vi "Final Labview.vi"() -> ()   [LabVIEW 2021]
panel:
  out "Ball 5 Color":string
  out "ball 4 y":dbl
  out "Ball 4 Color":string
  out "ball 3 x":dbl
  out "ball 4 x":dbl
  out "ball 3 y":dbl
  out "Ball 3 Color":string
  out "ball 2 y":dbl
  out "ball 5 x":dbl
  out "Ball 2 Color":string
  out "ball 5 y":dbl
  out "ball 2 x":dbl
  out "Ball 1 Color":string
  out "ball 1 y":dbl
  out "ball 1 x":dbl
  in  "Display History":bool
  out "2D Picture":picture
  in  "Size of Rectangle":i16
  out "y2":dbl=769.0125 format="%#.9g"
  out "x2":dbl=769.0125 format="%#.9g"
  out "y1":dbl=769.0125 format="%#.9g"
  out "x1":dbl=769.0125 format="%#.9g"
  out "Color":dbl=769.0125 format="%#.9g"
  out "Case Number":dbl=769.0125 format="%#.9g"
  out "Y":dbl=769.0125 format="%#.9g"
  out "X":dbl=769.0125 format="%#.9g"
  in  "Input 8":dbl=769.0125 format="%#.9g"
  in  "Input 7":dbl=769.0125 format="%#.9g"
  in  "Input 6":dbl=769.0125 format="%#.9g"
  in  "Input 5":dbl=769.0125 format="%#.9g"
  in  "Input 4":dbl=769.0125 format="%#.9g"
  in  "Input 3":dbl=769.0125 format="%#.9g"
  in  "Input 2":dbl=769.0125 format="%#.9g"
  in  "Input":dbl=769.0125 format="%#.9g"
  in  "stop":bool
  in  "SEND Button":bool
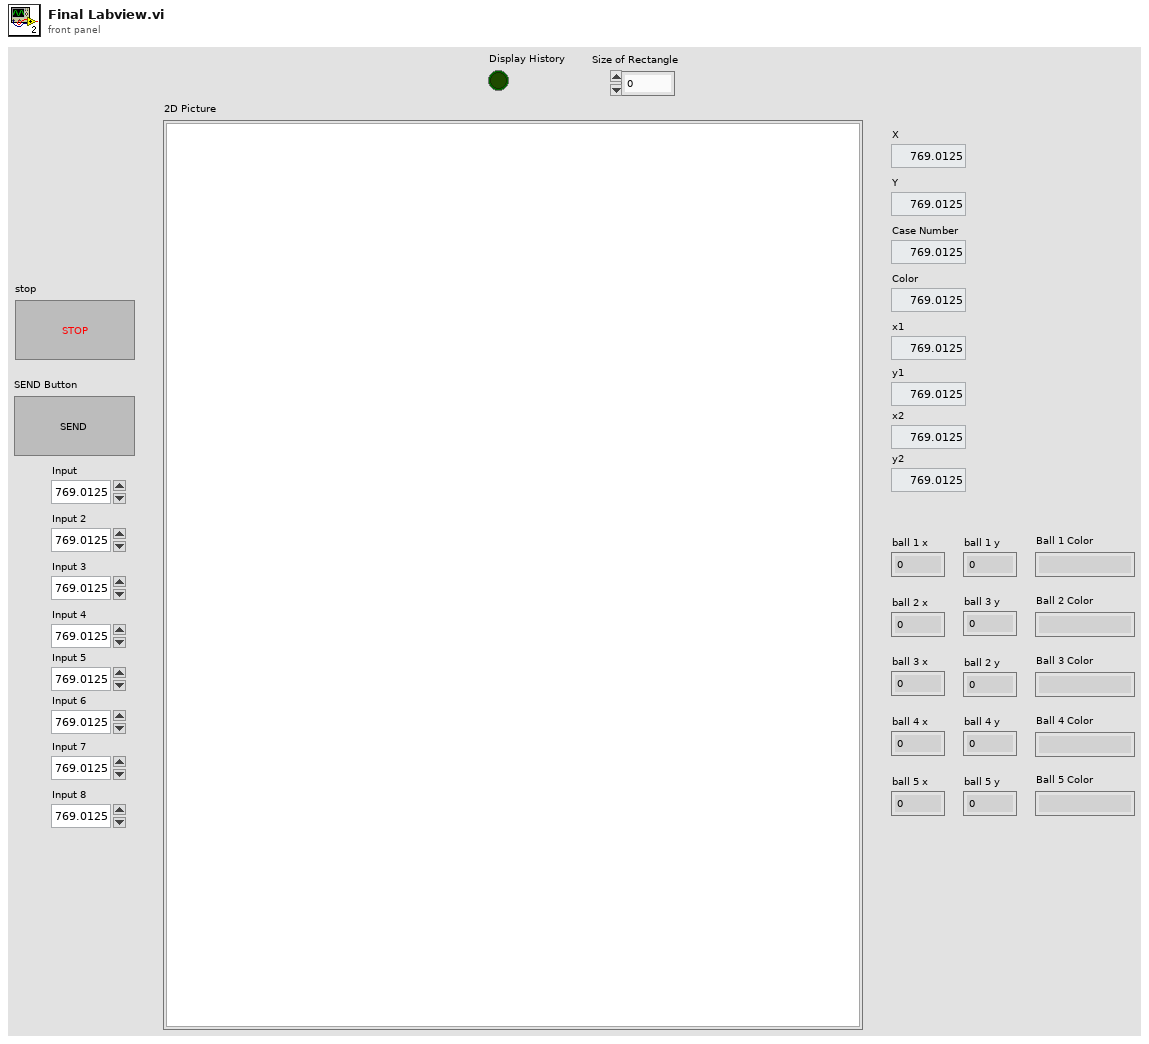
[diagram p1: front panel]
types:
  T1 = enum16{"Standard", "Buffered", "CRLF", "Immediate"}
  T2 = cluster{"Width":u16, "Style":enum32{"Solid", "Dash", "Dot", "DashDot", "DashDotDot"}}
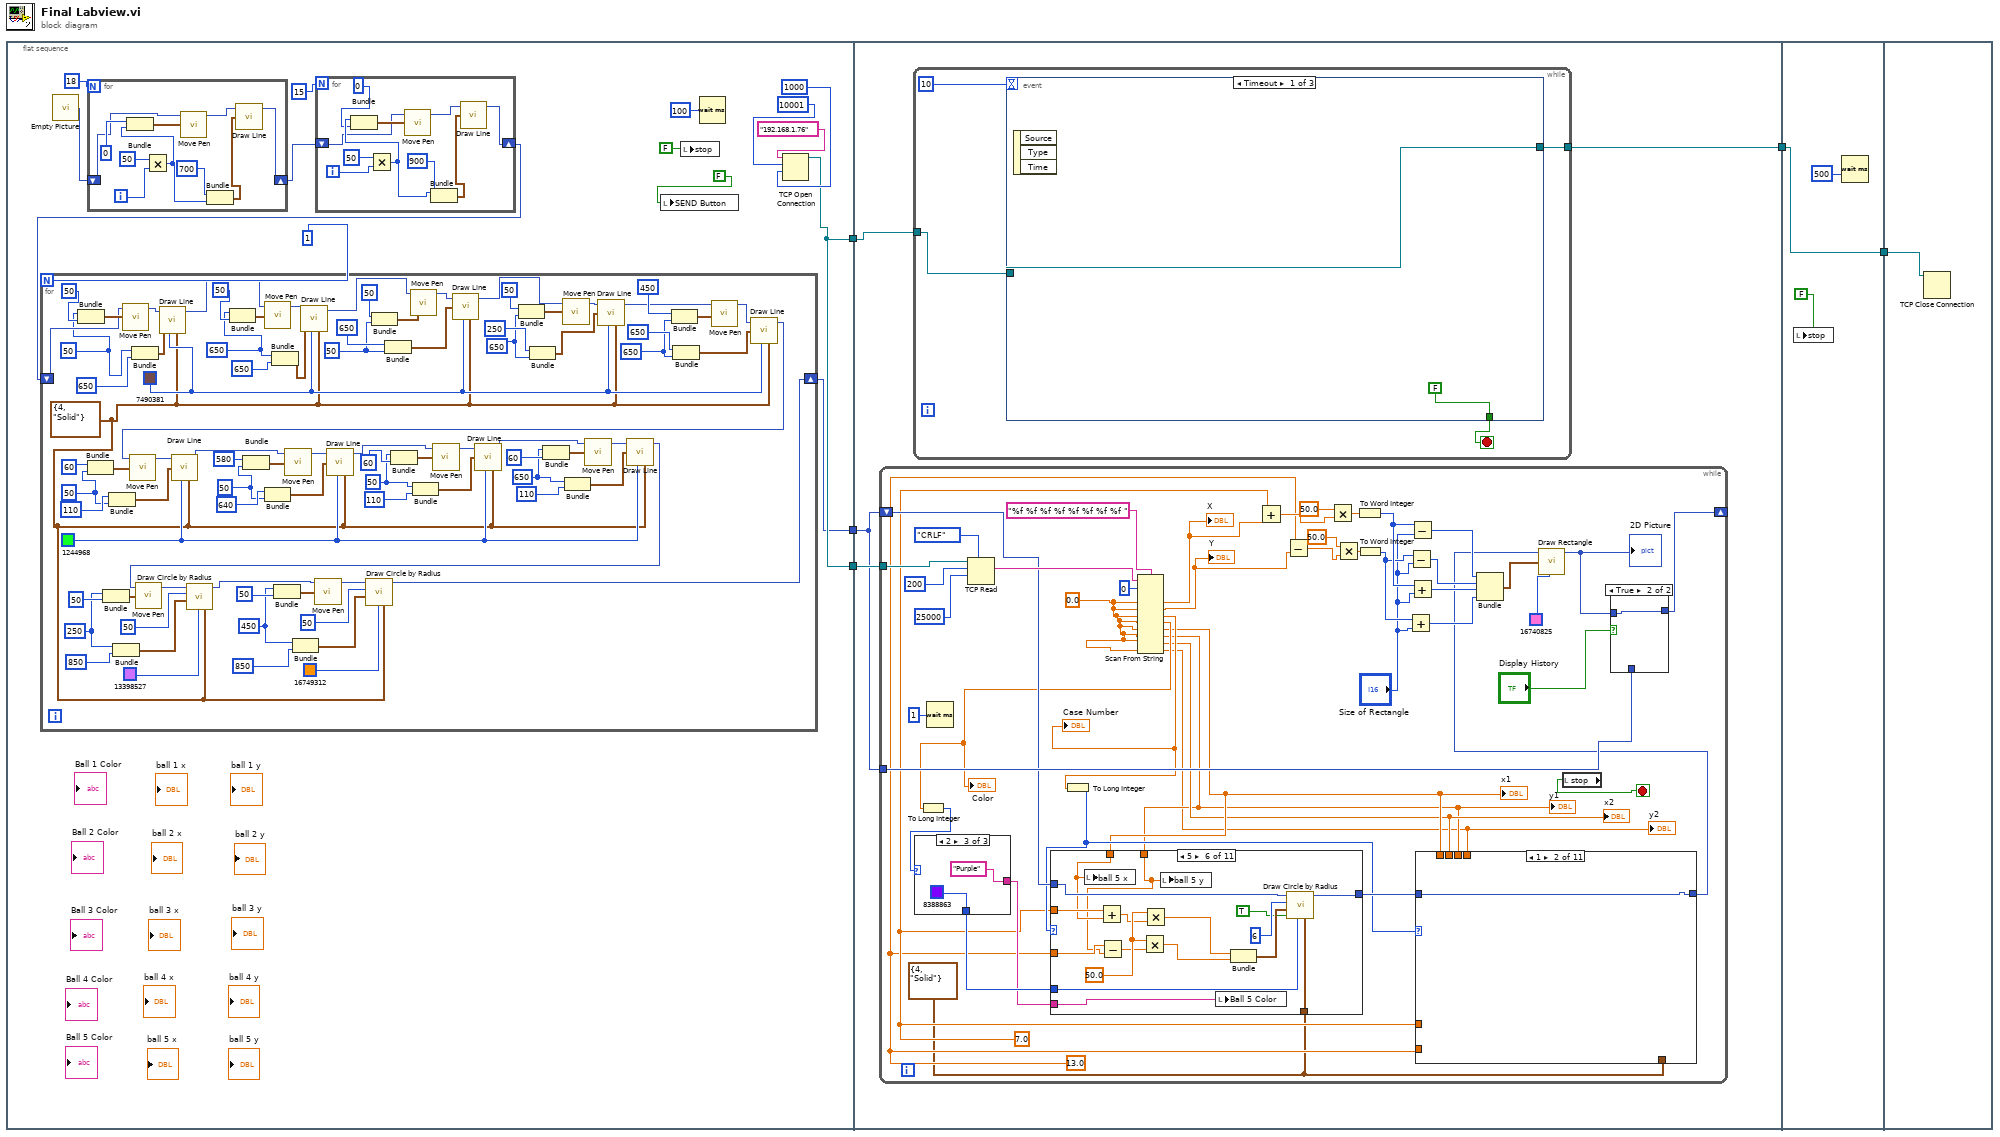
[diagram p0: block diagram]
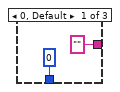
[diagram p2: hidden frame]
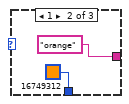
[diagram p3: hidden frame]
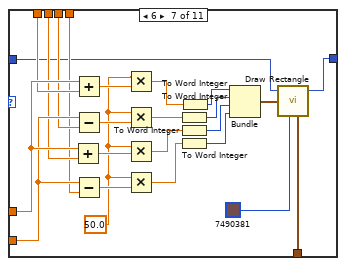
[diagram p9: hidden frame]
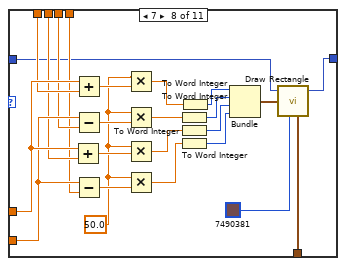
[diagram p10: hidden frame]
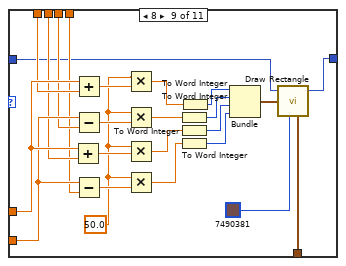
[diagram p11: hidden frame]
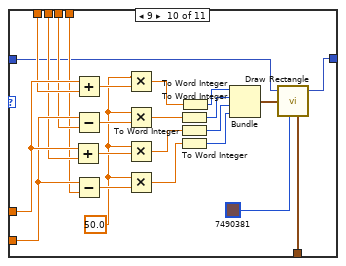
[diagram p12: hidden frame]
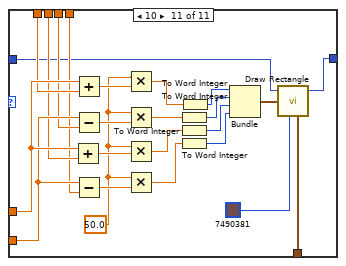
[diagram p13: hidden frame]
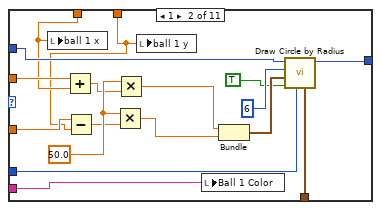
[diagram p15: hidden frame]
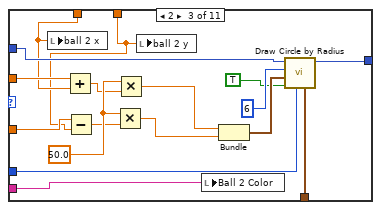
[diagram p16: hidden frame]
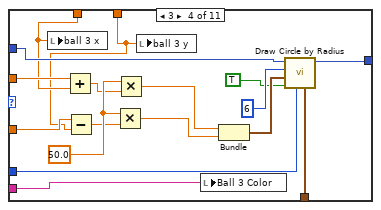
[diagram p17: hidden frame]
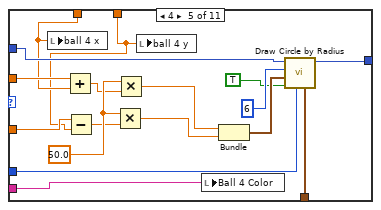
[diagram p18: hidden frame]
diagram:
  n1 = flat-sequence {
    tunnel: [w13] -> w5
    tunnel: [w13] -> w2
    tunnel: [w6] -> w1
    tunnel: w5 -> [w128]
    tunnel: [w127] -> w3
    tunnel: w2 -> [w126]
    tunnel: w1 -> [w125]
    tunnel: [w428] -> w4
    tunnel: w3 -> [w428]
    tunnel: w4 -> [w429]
    frame #0 {
      n2 = call "Empty Picture"() -> ("empty picture"=w9:picture)
      n3 = for {
        N: 18 -> [_]
        shift-right: [w115] -> w11
        shift-left: w9 -> [w116]
        i -> [w123]
        n4 = Multiply(x=50, y=w123) -> (x*y=w119:i32)
        n5 = Bundle(0, w119) -> (w120:cluster{i32, i32})  [unwired: 1 in]
        n6 = call <vilib>:"Move Pen.vi"("new position"=w120, "picture"=w116) -> ("new picture"=w124:picture)  [unwired: 3 in]
        n7 = Bundle(700, w119) -> (w117:cluster{i32, i32})  [unwired: 1 in]
        n8 = call <vilib>:"Draw Line.vi"("picture"=w124, "end point"=w117) -> ("new picture"=w115:picture)  [unwired: 7 in]
      }
      n9 = for {
        N: 15 -> [_]
        shift-right: [w105] -> w7
        shift-left: w11 -> [w106]
        i -> [w113]
        n10 = Multiply(x=50, y=w113) -> (x*y=w108:i32)
        n11 = Bundle(w108, 0) -> (w111:cluster{i32, i32})  [unwired: 1 in]
        n12 = call <vilib>:"Move Pen.vi"("new position"=w111, "picture"=w106) -> ("new picture"=w114:picture)  [unwired: 3 in]
        n13 = Bundle(w108, 900) -> (w110:cluster{i32, i32})  [unwired: 1 in]
        n14 = call <vilib>:"Draw Line.vi"("picture"=w114, "end point"=w110) -> ("new picture"=w105:picture)  [unwired: 7 in]
      }
      n15 = for {
        N: 1 -> [_]
        shift-right: [w21] -> w6
        shift-left: w7 -> [w99]
        w24 = 450 ("x")
        w32 = 250 ("x")
        w40 = 650 ("x")
        w42 = 50 ("x")
        w57 = 50 ("x")
        w46 = u32 1244968 ("Hilite")
        w63 = 50 ("x")
        w69 = 650 ("x")
        w20 = T2 {"Width"=4, "Style"=enum."Solid"} ("pen")
        w70 = 650 ("x")
        w71 = 50 ("x")
        w72 = 650 ("x")
        w74 = u32 7490381 ("Hilite")
        w73 = 50 ("x")
        n16 = Bundle("x"=w73, 50) -> (w103:cluster{"x":i32, i32})  [unwired: 1 in]
        n17 = Bundle(60, "x"=w63) -> (w66:cluster{i32, "x":i32})  [unwired: 1 in]
        n18 = Bundle("x"=w32, 50) -> (w39:cluster{"x":i32, i32})  [unwired: 1 in]
        n19 = Bundle(110, "x"=w63) -> (w64:cluster{i32, "x":i32})  [unwired: 1 in]
        n20 = Bundle("x"=w32, 850) -> (w33:cluster{"x":i32, i32})  [unwired: 1 in]
        n21 = call <vilib>:"Move Pen.vi"("new position"=w103, "picture"=w99) -> ("new picture"=w104:picture)  [unwired: 3 in]
        n22 = Bundle("x"=w73, 650) -> (w102:cluster{"x":i32, i32})  [unwired: 1 in]
        n23 = call <vilib>:"Draw Line.vi"("picture"=w104, "end point"=w102, "color(black)"=w74, "pen"=w20) -> ("new picture"=w93:picture)  [unwired: 5 in]
        n24 = Bundle("x"=w72, 50) -> (w97:cluster{"x":i32, i32})  [unwired: 1 in]
        n25 = Bundle(580, "x"=w57) -> (w60:cluster{i32, "x":i32})  [unwired: 1 in]
        n26 = call <vilib>:"Move Pen.vi"("new position"=w97, "picture"=w93) -> ("new picture"=w98:picture)  [unwired: 3 in]
        n27 = Bundle(640, "x"=w57) -> (w58:cluster{i32, "x":i32})  [unwired: 1 in]
        n28 = Bundle("x"=w72, 650) -> (w96:cluster{"x":i32, i32})  [unwired: 1 in]
        n29 = Bundle("x"=w24, 50) -> (w31:cluster{"x":i32, i32})  [unwired: 1 in]
        n30 = Bundle("x"=w24, 850) -> (w25:cluster{"x":i32, i32})  [unwired: 1 in]
        n31 = call <vilib>:"Draw Line.vi"("picture"=w98, "end point"=w96, "color(black)"=w74, "pen"=w20) -> ("new picture"=w89:picture)  [unwired: 5 in]
        n32 = Bundle(50, "x"=w71) -> (w91:cluster{i32, "x":i32})  [unwired: 1 in]
        n33 = Bundle(650, "x"=w71) -> (w90:cluster{i32, "x":i32})  [unwired: 1 in]
        n34 = Bundle("x"=w42, 60) -> (w55:cluster{"x":i32, i32})  [unwired: 1 in]
        n35 = call <vilib>:"Move Pen.vi"("new position"=w91, "picture"=w89) -> ("new picture"=w92:picture)  [unwired: 3 in]
        n36 = Bundle("x"=w42, 110) -> (w54:cluster{"x":i32, i32})  [unwired: 1 in]
        n37 = call <vilib>:"Draw Line.vi"("picture"=w92, "end point"=w90, "color(black)"=w74, "pen"=w20) -> ("new picture"=w84:picture)  [unwired: 5 in]
        n38 = Bundle(50, "x"=w70) -> (w86:cluster{i32, "x":i32})  [unwired: 1 in]
        n39 = Bundle(250, "x"=w70) -> (w85:cluster{i32, "x":i32})  [unwired: 1 in]
        n40 = Bundle("x"=w40, 60) -> (w52:cluster{"x":i32, i32})  [unwired: 1 in]
        n41 = call <vilib>:"Move Pen.vi"("new position"=w86, "picture"=w84) -> ("new picture"=w87:picture)  [unwired: 3 in]
        n42 = Bundle("x"=w40, 110) -> (w51:cluster{"x":i32, i32})  [unwired: 1 in]
        n43 = call <vilib>:"Draw Line.vi"("picture"=w87, "end point"=w85, "color(black)"=w74, "pen"=w20) -> ("new picture"=w75:picture)  [unwired: 5 in]
        n44 = Bundle(450, "x"=w69) -> (w79:cluster{i32, "x":i32})  [unwired: 1 in]
        n45 = Bundle(650, "x"=w69) -> (w78:cluster{i32, "x":i32})  [unwired: 1 in]
        n46 = call <vilib>:"Move Pen.vi"("new position"=w79, "picture"=w75) -> ("new picture"=w80:picture)  [unwired: 3 in]
        n47 = call <vilib>:"Draw Line.vi"("picture"=w80, "end point"=w78, "color(black)"=w74, "pen"=w20) -> ("new picture"=w50:picture)  [unwired: 5 in]
        n48 = call <vilib>:"Move Pen.vi"("new position"=w66, "picture"=w50) -> ("new picture"=w68:picture)  [unwired: 3 in]
        n49 = call <vilib>:"Draw Line.vi"("picture"=w68, "end point"=w64, "color(black)"=w46, "pen"=w20) -> ("new picture"=w49:picture)  [unwired: 5 in]
        n50 = call <vilib>:"Move Pen.vi"("new position"=w60, "picture"=w49) -> ("new picture"=w62:picture)  [unwired: 3 in]
        n51 = call <vilib>:"Draw Line.vi"("picture"=w62, "end point"=w58, "color(black)"=w46, "pen"=w20) -> ("new picture"=w48:picture)  [unwired: 5 in]
        n52 = call <vilib>:"Move Pen.vi"("new position"=w55, "picture"=w48) -> ("new picture"=w56:picture)  [unwired: 3 in]
        n53 = call <vilib>:"Draw Line.vi"("picture"=w56, "end point"=w54, "color(black)"=w46, "pen"=w20) -> ("new picture"=w47:picture)  [unwired: 5 in]
        n54 = call <vilib>:"Move Pen.vi"("new position"=w52, "picture"=w47) -> ("new picture"=w53:picture)  [unwired: 3 in]
        n55 = call <vilib>:"Draw Line.vi"("picture"=w53, "end point"=w51, "color(black)"=w46, "pen"=w20) -> ("new picture"=w23:picture)  [unwired: 5 in]
        n56 = call <vilib>:"Move Pen.vi"("new position"=w39, "picture"=w23) -> ("new picture"=w36:picture)  [unwired: 3 in]
        n57 = call <vilib>:"Draw Circle by Radius.vi"("pen"=w20, "color(black)"=u32 13398527 ("Hilite"), "pixel center"=w33, "radius"=i16 50, "picture"=w36) -> ("new picture"=w22:picture)  [unwired: 6 in]
        n58 = call <vilib>:"Move Pen.vi"("new position"=w31, "picture"=w22) -> ("new picture"=w28:picture)  [unwired: 3 in]
        n59 = call <vilib>:"Draw Circle by Radius.vi"("pen"=w20, "color(black)"=u32 16749312 ("Hilite"), "pixel center"=w25, "radius"=i16 50, "picture"=w28) -> ("new picture"=w21:picture)  [unwired: 6 in]
      }
      n60 = local write "SEND Button"(FALSE ("SEND Button")) -> ()
      n61 = local write "stop"(FALSE ("stop")) -> ()
      n62 = Wait (ms)(milliseconds to wait=u32 100) -> ()  [unwired: 1 out]
      n63 = TCP Open Connection(address="192.168.1.76", remote port or service name=u16 10001, timeout ms (60000)=1000) -> (connection ID=w13:refnum<k5>)  [unwired: 2 in, 1 out]
    }
    frame #1 {
      n64 = while {
        tunnel: w126 -> [w158]
        tunnel: w125 -> [w146]
        shift-right: [w155] -> _
        shift-left: w125 -> [w141]
        stop <- w147 stop-if-true
        w129 = T2 {"Width"=4, "Style"=enum."Solid"} ("pen")
        w134 = 13.0 ("x")
        w135 = 7.0 ("x")
        w145 = 0.0 ("default value 1")
        n65 = Wait (ms)(milliseconds to wait=u32 1) -> ()  [unwired: 1 out]
        n66 = TCP Read(connection ID=w158, bytes to read=200, 7:T1."CRLF" ("mode (standard)"), 9:25000 ("timeout ms (25000)")) -> (data out=w170:string)  [unwired: 1 in, 2 out]
        n67 = Scan From String(format string="%f %f %f %f %f %f %f %f ", input string=w170, initial scan location=u32 0, default 1=w145, default 2=w145, default 3=w145, default 4=w145, default 5=w145, default 6=w145, default 7=w145, default 8=w145) -> (output 1=w169:dbl, output 2=w168:dbl, output 3=w144:dbl, output 4=w138:dbl, output 5=w133:dbl, output 6=w131:dbl, output 7=w132:dbl, output 8=w130:dbl)  [unwired: 1 in, 3 out]
        "X" <- w169
        "Y" <- w168
        "Case Number" <- w144
        "Color" <- w138
        "x1" <- w133
        "y1" <- w131
        "x2" <- w132
        "y2" <- w130
        n68 = To Long Integer(number=w138) -> (32bit integer=w137:i32)
        n69 = case shown="2" w137 {
          tunnel: [u32 0 ("Hilite") u32 16749312 ("Hilite") u32 8388863 ("Hilite")] -> w143
          tunnel: ["" ("color 1") "orange" ("color 1") "Purple" ("color 1")] -> w142
          frame 0, Default {
          }
          frame 1 {
          }
          frame 2 {
          }
        }
        n70 = To Long Integer(number=w144) -> (32bit integer=w136:i32)
        n71 = case shown="5" w136 {
          tunnel: w141 -> [w308 w319 w336 w353 w370 w387 w394 w395 w396 w397 w398]
          tunnel: w131 -> [_ w313 w330 w347 w364 w381 _ _ _ _ _]
          tunnel: w133 -> [_ w314 w331 w348 w365 w382 _ _ _ _ _]
          tunnel: w129 -> [_ w322 w339 w356 w373 w390 _ _ _ _ _]
          tunnel: w143 -> [_ w321 w338 w355 w372 w389 _ _ _ _ _]
          tunnel: w142 -> [_ w320 w337 w354 w371 w388 _ _ _ _ _]
          tunnel: [w308 w318 w335 w352 w369 w386 w394 w395 w396 w397 w398] -> w140
          tunnel: w135 -> [_ w316 w333 w350 w367 w384 _ _ _ _ _]
          tunnel: w134 -> [_ w315 w332 w349 w366 w383 _ _ _ _ _]
          frame 0, Default {
          }
          frame 1 {
            w317 = 50.0 ("x")
            n72 = local write "ball 1 x"(w314) -> ()
            n73 = Add(x=w316, y=w314) -> (x+y=w312:dbl)
            n74 = Subtract(x=w315, y=w313) -> (x-y=w311:dbl)
            n75 = Multiply(x=w317, y=w311) -> (x*y=w309:dbl)
            n76 = Multiply(x=w317, y=w312) -> (x*y=w310:dbl)
            n77 = local write "ball 1 y"(w313) -> ()
            n78 = local write "Ball 1 Color"(w320) -> ()
            n79 = Bundle(w310, w309) -> (w324:cluster{dbl, dbl})  [unwired: 1 in]
            n80 = call <vilib>:"Draw Circle by Radius.vi"("pen"=w322, "color(black)"=w321, "fill?(F)"=TRUE, "pixel center"=w324, "radius"=i16 6, "picture"=w319) -> ("new picture"=w318:picture)  [unwired: 5 in]
          }
          frame 2 {
            w334 = 50.0 ("x")
            n81 = local write "ball 2 x"(w331) -> ()
            n82 = Add(x=w333, y=w331) -> (x+y=w329:dbl)
            n83 = Subtract(x=w332, y=w330) -> (x-y=w328:dbl)
            n84 = Multiply(x=w334, y=w328) -> (x*y=w326:dbl)
            n85 = Multiply(x=w334, y=w329) -> (x*y=w327:dbl)
            n86 = local write "ball 2 y"(w330) -> ()
            n87 = local write "Ball 2 Color"(w337) -> ()
            n88 = Bundle(w327, w326) -> (w341:cluster{dbl, dbl})  [unwired: 1 in]
            n89 = call <vilib>:"Draw Circle by Radius.vi"("pen"=w339, "color(black)"=w338, "fill?(F)"=TRUE, "pixel center"=w341, "radius"=i16 6, "picture"=w336) -> ("new picture"=w335:picture)  [unwired: 5 in]
          }
          frame 3 {
            w351 = 50.0 ("x")
            n90 = local write "ball 3 x"(w348) -> ()
            n91 = Add(x=w350, y=w348) -> (x+y=w346:dbl)
            n92 = Subtract(x=w349, y=w347) -> (x-y=w345:dbl)
            n93 = Multiply(x=w351, y=w345) -> (x*y=w343:dbl)
            n94 = Multiply(x=w351, y=w346) -> (x*y=w344:dbl)
            n95 = local write "ball 3 y"(w347) -> ()
            n96 = local write "Ball 3 Color"(w354) -> ()
            n97 = Bundle(w344, w343) -> (w358:cluster{dbl, dbl})  [unwired: 1 in]
            n98 = call <vilib>:"Draw Circle by Radius.vi"("pen"=w356, "color(black)"=w355, "fill?(F)"=TRUE, "pixel center"=w358, "radius"=i16 6, "picture"=w353) -> ("new picture"=w352:picture)  [unwired: 5 in]
          }
          frame 4 {
            w368 = 50.0 ("x")
            n99 = local write "ball 4 x"(w365) -> ()
            n100 = Add(x=w367, y=w365) -> (x+y=w363:dbl)
            n101 = Subtract(x=w366, y=w364) -> (x-y=w362:dbl)
            n102 = Multiply(x=w368, y=w362) -> (x*y=w360:dbl)
            n103 = Multiply(x=w368, y=w363) -> (x*y=w361:dbl)
            n104 = local write "ball 4 y"(w364) -> ()
            n105 = local write "Ball 4 Color"(w371) -> ()
            n106 = Bundle(w361, w360) -> (w375:cluster{dbl, dbl})  [unwired: 1 in]
            n107 = call <vilib>:"Draw Circle by Radius.vi"("pen"=w373, "color(black)"=w372, "fill?(F)"=TRUE, "pixel center"=w375, "radius"=i16 6, "picture"=w370) -> ("new picture"=w369:picture)  [unwired: 5 in]
          }
          frame 5 {
            w385 = 50.0 ("x")
            n108 = local write "ball 5 x"(w382) -> ()
            n109 = Add(x=w384, y=w382) -> (x+y=w380:dbl)
            n110 = Subtract(x=w383, y=w381) -> (x-y=w379:dbl)
            n111 = Multiply(x=w385, y=w379) -> (x*y=w377:dbl)
            n112 = Multiply(x=w385, y=w380) -> (x*y=w378:dbl)
            n113 = local write "ball 5 y"(w381) -> ()
            n114 = local write "Ball 5 Color"(w388) -> ()
            n115 = Bundle(w378, w377) -> (w392:cluster{dbl, dbl})  [unwired: 1 in]
            n116 = call <vilib>:"Draw Circle by Radius.vi"("pen"=w390, "color(black)"=w389, "fill?(F)"=TRUE, "pixel center"=w392, "radius"=i16 6, "picture"=w387) -> ("new picture"=w386:picture)  [unwired: 5 in]
          }
          frame 6 {
          }
          frame 7 {
          }
          frame 8 {
          }
          frame 9 {
          }
          frame 10 {
          }
        }
        n117 = Add(x=w135, y=w169) -> (x+y=w165:dbl)
        n118 = Subtract(x=w134, y=w168) -> (x-y=w164:dbl)
        n119 = Multiply(x=50.0, y=w165) -> (x*y=w162:dbl)
        n120 = Multiply(x=50.0, y=w164) -> (x*y=w163:dbl)
        n121 = To Word Integer(number=w162) -> (16bit integer=w161:i16)
        n122 = To Word Integer(number=w163) -> (16bit integer=w160:i16)
        n123 = Add(x=w160, y="Size of Rectangle") -> (x+y=w151:i16)
        n124 = Subtract(x=w160, y="Size of Rectangle") -> (x-y=w153:i16)
        n125 = Subtract(x=w161, y="Size of Rectangle") -> (x-y=w154:i16)
        n126 = Add(x=w161, y="Size of Rectangle") -> (x+y=w152:i16)
        n127 = case shown="1" w136 {
          tunnel: w140 -> [w182 w183 w184 w185 w186 w187 w196 w220 w244 w268 w292]
          tunnel: [w182 w183 w184 w185 w186 w187 w190 w214 w238 w262 w286] -> w139
          tunnel: w135 -> [_ _ _ _ _ _ w211 w235 w259 w283 w307]
          tunnel: w134 -> [_ _ _ _ _ _ w210 w234 w258 w282 w306]
          tunnel: w133 -> [_ _ _ _ _ _ w209 w233 w257 w281 w305]
          tunnel: w132 -> [_ _ _ _ _ _ w208 w232 w256 w280 w304]
          tunnel: w131 -> [_ _ _ _ _ _ w207 w231 w255 w279 w303]
          tunnel: w130 -> [_ _ _ _ _ _ w206 w230 w254 w278 w302]
          tunnel: w129 -> [_ _ _ _ _ _ w188 w212 w236 w260 w284]
          frame 0, Default {
          }
          frame 1 {
          }
          frame 2 {
          }
          frame 3 {
          }
          frame 4 {
          }
          frame 5 {
          }
          frame 6 {
            w201 = 50.0 ("x")
            n128 = Add(x=w211, y=w208) -> (x+y=w203:dbl)
            n129 = Add(x=w211, y=w209) -> (x+y=w205:dbl)
            n130 = Subtract(x=w210, y=w207) -> (x-y=w204:dbl)
            n131 = Subtract(x=w210, y=w206) -> (x-y=w202:dbl)
            n132 = Multiply(x=w201, y=w205) -> (x*y=w200:dbl)
            n133 = Multiply(x=w201, y=w204) -> (x*y=w199:dbl)
            n134 = Multiply(x=w201, y=w203) -> (x*y=w198:dbl)
            n135 = Multiply(x=w201, y=w202) -> (x*y=w197:dbl)
            n136 = To Word Integer(number=w199) -> (16bit integer=w194:i16)
            n137 = To Word Integer(number=w198) -> (16bit integer=w193:i16)
            n138 = To Word Integer(number=w197) -> (16bit integer=w192:i16)
            n139 = To Word Integer(number=w200) -> (16bit integer=w195:i16)
            n140 = Bundle(w195, w194, w193, w192) -> (w191:cluster{i16, i16, i16, i16})  [unwired: 1 in]
            n141 = call <vilib>:"Draw Rectangle.vi"("picture"=w196, "rect"=w191, "color(black)"=u32 7490381 ("Hilite"), "pen"=w188) -> ("new picture"=w190:picture)  [unwired: 5 in]
          }
          frame 7 {
            w225 = 50.0 ("x")
            n142 = Add(x=w235, y=w232) -> (x+y=w227:dbl)
            n143 = Add(x=w235, y=w233) -> (x+y=w229:dbl)
            n144 = Subtract(x=w234, y=w231) -> (x-y=w228:dbl)
            n145 = Subtract(x=w234, y=w230) -> (x-y=w226:dbl)
            n146 = Multiply(x=w225, y=w229) -> (x*y=w224:dbl)
            n147 = Multiply(x=w225, y=w228) -> (x*y=w223:dbl)
            n148 = Multiply(x=w225, y=w227) -> (x*y=w222:dbl)
            n149 = Multiply(x=w225, y=w226) -> (x*y=w221:dbl)
            n150 = To Word Integer(number=w223) -> (16bit integer=w218:i16)
            n151 = To Word Integer(number=w222) -> (16bit integer=w217:i16)
            n152 = To Word Integer(number=w221) -> (16bit integer=w216:i16)
            n153 = To Word Integer(number=w224) -> (16bit integer=w219:i16)
            n154 = Bundle(w219, w218, w217, w216) -> (w215:cluster{i16, i16, i16, i16})  [unwired: 1 in]
            n155 = call <vilib>:"Draw Rectangle.vi"("picture"=w220, "rect"=w215, "color(black)"=u32 7490381 ("Hilite"), "pen"=w212) -> ("new picture"=w214:picture)  [unwired: 5 in]
          }
          frame 8 {
            w249 = 50.0 ("x")
            n156 = Add(x=w259, y=w256) -> (x+y=w251:dbl)
            n157 = Add(x=w259, y=w257) -> (x+y=w253:dbl)
            n158 = Subtract(x=w258, y=w255) -> (x-y=w252:dbl)
            n159 = Subtract(x=w258, y=w254) -> (x-y=w250:dbl)
            n160 = Multiply(x=w249, y=w253) -> (x*y=w248:dbl)
            n161 = Multiply(x=w249, y=w252) -> (x*y=w247:dbl)
            n162 = Multiply(x=w249, y=w251) -> (x*y=w246:dbl)
            n163 = Multiply(x=w249, y=w250) -> (x*y=w245:dbl)
            n164 = To Word Integer(number=w247) -> (16bit integer=w242:i16)
            n165 = To Word Integer(number=w246) -> (16bit integer=w241:i16)
            n166 = To Word Integer(number=w245) -> (16bit integer=w240:i16)
            n167 = To Word Integer(number=w248) -> (16bit integer=w243:i16)
            n168 = Bundle(w243, w242, w241, w240) -> (w239:cluster{i16, i16, i16, i16})  [unwired: 1 in]
            n169 = call <vilib>:"Draw Rectangle.vi"("picture"=w244, "rect"=w239, "color(black)"=u32 7490381 ("Hilite"), "pen"=w236) -> ("new picture"=w238:picture)  [unwired: 5 in]
          }
          frame 9 {
            w273 = 50.0 ("x")
            n170 = Add(x=w283, y=w280) -> (x+y=w275:dbl)
            n171 = Add(x=w283, y=w281) -> (x+y=w277:dbl)
            n172 = Subtract(x=w282, y=w279) -> (x-y=w276:dbl)
            n173 = Subtract(x=w282, y=w278) -> (x-y=w274:dbl)
            n174 = Multiply(x=w273, y=w277) -> (x*y=w272:dbl)
            n175 = Multiply(x=w273, y=w276) -> (x*y=w271:dbl)
            n176 = Multiply(x=w273, y=w275) -> (x*y=w270:dbl)
            n177 = Multiply(x=w273, y=w274) -> (x*y=w269:dbl)
            n178 = To Word Integer(number=w271) -> (16bit integer=w266:i16)
            n179 = To Word Integer(number=w270) -> (16bit integer=w265:i16)
            n180 = To Word Integer(number=w269) -> (16bit integer=w264:i16)
            n181 = To Word Integer(number=w272) -> (16bit integer=w267:i16)
            n182 = Bundle(w267, w266, w265, w264) -> (w263:cluster{i16, i16, i16, i16})  [unwired: 1 in]
            n183 = call <vilib>:"Draw Rectangle.vi"("picture"=w268, "rect"=w263, "color(black)"=u32 7490381 ("Hilite"), "pen"=w260) -> ("new picture"=w262:picture)  [unwired: 5 in]
          }
          frame 10 {
            w297 = 50.0 ("x")
            n184 = Add(x=w307, y=w304) -> (x+y=w299:dbl)
            n185 = Add(x=w307, y=w305) -> (x+y=w301:dbl)
            n186 = Subtract(x=w306, y=w303) -> (x-y=w300:dbl)
            n187 = Subtract(x=w306, y=w302) -> (x-y=w298:dbl)
            n188 = Multiply(x=w297, y=w301) -> (x*y=w296:dbl)
            n189 = Multiply(x=w297, y=w300) -> (x*y=w295:dbl)
            n190 = Multiply(x=w297, y=w299) -> (x*y=w294:dbl)
            n191 = Multiply(x=w297, y=w298) -> (x*y=w293:dbl)
            n192 = To Word Integer(number=w295) -> (16bit integer=w290:i16)
            n193 = To Word Integer(number=w294) -> (16bit integer=w289:i16)
            n194 = To Word Integer(number=w293) -> (16bit integer=w288:i16)
            n195 = To Word Integer(number=w296) -> (16bit integer=w291:i16)
            n196 = Bundle(w291, w290, w289, w288) -> (w287:cluster{i16, i16, i16, i16})  [unwired: 1 in]
            n197 = call <vilib>:"Draw Rectangle.vi"("picture"=w292, "rect"=w287, "color(black)"=u32 7490381 ("Hilite"), "pen"=w284) -> ("new picture"=w286:picture)  [unwired: 5 in]
          }
        }
        n198 = Bundle(w154, w153, w152, w151) -> (w148:cluster{i16, i16, i16, i16})  [unwired: 1 in]
        n199 = call <vilib>:"Draw Rectangle.vi"("picture"=w139, "rect"=w148, "color(black)"=u32 16740825) -> ("new picture"=w150:picture)  [unwired: 6 in]
        "2D Picture" <- w150
        n200 = local read "stop"() -> (w147:bool)
        n201 = case shown="True" "Display History" {
          tunnel: [w399 w400] -> w155
          tunnel: w150 -> [_ w400]
          tunnel: w146 -> [w399 _]
          frame False {
          }
          frame True {
          }
        }
      }
      n202 = while {
        tunnel: w128 -> [w404]
        tunnel: [w403] -> w127
        stop <- w402 stop-if-true
        n203 = event shown="[0] Timeout" {
          selector: _ -> [_ _ _]
          dyn-events: _ -> [_ _ _]
          timeout: 10 -> [_ _ _]
          tunnel: w404 -> [w405 w407 w411]
          tunnel: [w405 w407 w410] -> w403
          tunnel: [FALSE TRUE FALSE] -> w402
          event Timeout {
            n204 = event-data() -> ()  [unwired: 1 in, 3 out]
          }
          event "stop": Value Change {
            n205 = event-data() -> ()  [unwired: 1 in, 6 out]
          }
          event "SEND Button": Value Change {
            n206 = event-data() -> ()  [unwired: 1 in, 6 out]
            n207 = Format Into String(format string="%f %f %f %f %f %f %f %f ", "Input", "Input 2", "Input 3", "Input 4", "Input 5", "Input 6", "Input 7", "Input 8") -> (resulting string=w414:string)  [unwired: 2 in, 1 out]
            n208 = Concatenate Strings("ý" ("string"), w414, "ÿ" ("string")) -> (w415:string)
            n209 = TCP Write(connection ID=w411, data in=w415, 9:100 ("timeout ms (25000)")) -> (connection ID out=w410:refnum<k5>)  [unwired: 1 in, 2 out]
          }
        }
      }
    }
    frame #2 {
      n210 = local write "stop"(FALSE) -> ()
      n211 = Wait (ms)(milliseconds to wait=u32 500) -> ()  [unwired: 1 out]
    }
    frame #3 {
      n212 = TCP Close Connection(connection ID=w429) -> ()  [unwired: 2 in, 2 out]
    }
  }
